vi "BusB Decoded Data Updated.vi"(8 "error in (no error)":errorcluster, 11 "BusB TypeDef":T1) -> (0 "error out":errorcluster)   [LabVIEW 2016, in "Impedance Data Acquisition and Decoding.lvlib"]
doc: "_____\nCreated using Delacor QMH Event Scripter 5.0.0.112."
uses:
  Impedance Data Acquisition and Decoding.lvlib
  BusB Typedef.ctl
  BusB Decoded Data Updated Argument--cluster.ctl
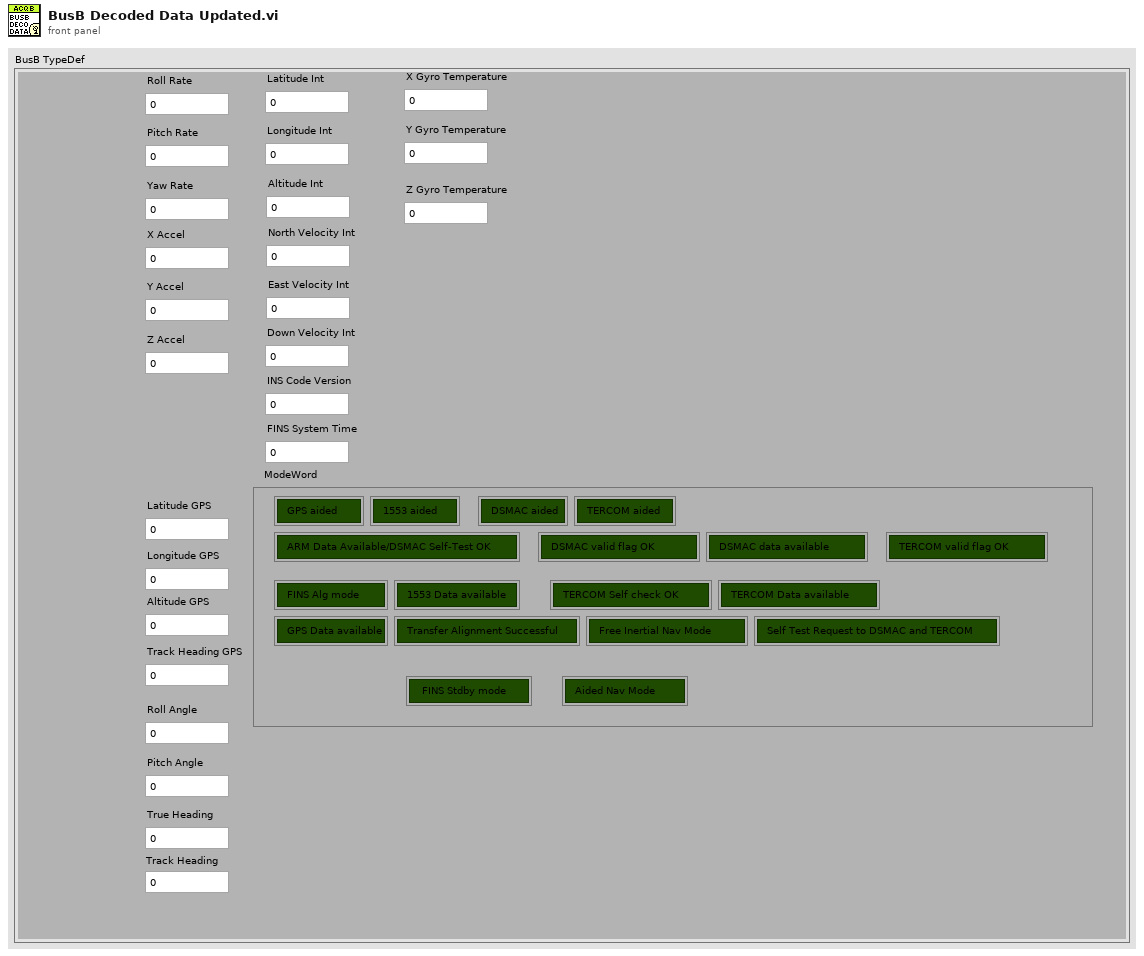
[diagram p1: front panel]
types:
  T1 = typedef "Impedance Data Acquisition and Decoding.lvlib/BusB Typedef.ctl" = cluster{"Pitch Rate":dbl, "Roll Rate":dbl, "Roll Angle":dbl, "Yaw Rate":dbl, "True Heading":dbl, "Pitch Angle":dbl, "Y Accel":dbl, "X Accel":dbl, "Z Accel":dbl, "X Gyro Temperature":dbl, "Longitude GPS":dbl, "Latitude GPS":dbl, "Altitude GPS":dbl, "Track Heading GPS":dbl, "Longitude Int":dbl, "Latitude Int":dbl, "Altitude Int":dbl, "FINS System Time":dbl, "East Velocity Int":dbl, "North Velocity Int":dbl, "INS Code Version":dbl, "ModeWord":cluster{"FINS Alg mode":bool, "GPS Data available":bool, "1553 Data available":bool, "Transfer Alignment Successful":bool, "TERCOM Self check OK":bool, "Free Inertial Nav Mode":bool, "TERCOM Data available":bool, "Self Test Request to DSMAC and TERCOM":bool, "ARM Data Available/DSMAC Self-Test OK":bool, "DSMAC valid flag OK":bool, "DSMAC data available":bool, "TERCOM valid flag OK":bool, "GPS aided":bool, "1553 aided":bool, "DSMAC aided":bool, "TERCOM aided":bool, "Aided Nav Mode":bool, " FINS Stdby mode":bool}, "Down Velocity Int":dbl, "Track Heading":dbl, "Y Gyro Temperature":dbl, "Z Gyro Temperature":dbl}
  T2 = typedef "Impedance Data Acquisition and Decoding.lvlib/BusB Decoded Data Updated Argument--cluster.ctl" = cluster{"BusB Decoded Data":T1}
  T3 = typedef "Impedance Data Acquisition and Decoding.lvlib/Broadcast Events--cluster.ctl" = cluster{"Module Did Init":refnum<user-event>, "Status Updated":refnum<user-event>, "Error Reported":refnum<user-event>, "Module Did Stop":refnum<user-event>, "Update Module Execution Status":refnum<user-event>, "Acquisition Stopped":refnum<user-event>, "BusB Raw Data":refnum<user-event>, "BusB Decoded Data Updated":refnum<user-event>, "Acquisition Started":refnum<user-event>, "Read Timeout Error Generation":refnum<user-event>}
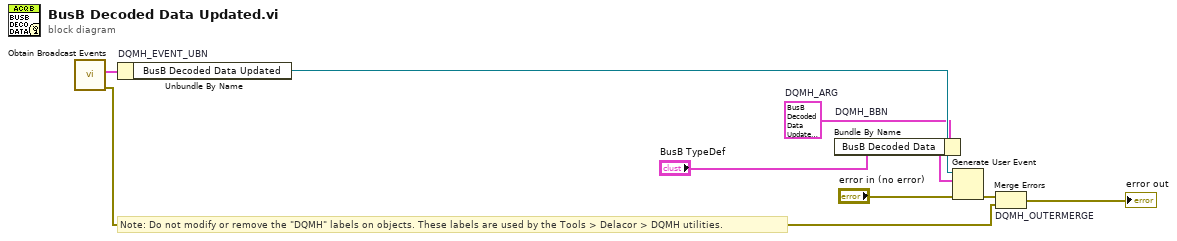
[diagram p0: block diagram]
diagram:
  w4 = T2 {"BusB Decoded Data"={"Pitch Rate"=0.0, "Roll Rate"=0.0, "Roll Angle"=0.0, "Yaw Rate"=0.0, "True Heading"=0.0, "Pitch Angle"=0.0, "Y Accel"=0.0, "X Accel"=0.0, "Z Accel"=0.0, "X Gyro Temperature"=0.0, "Longitude GPS"=0.0, "Latitude GPS"=0.0, "Altitude GPS"=0.0, "Track Heading GPS"=0.0, "Longitude Int"=0.0, "Latitude Int"=0.0, "Altitude Int"=0.0, "FINS System Time"=0.0, "East Velocity Int"=0.0, "North Velocity Int"=0.0, "INS Code Version"=0.0, "ModeWord"={"FINS Alg mode"=FALSE, "GPS Data available"=FALSE, "1553 Data available"=FALSE, "Transfer Alignment Successful"=FALSE, "TERCOM Self check OK"=FALSE, "Free Inertial Nav Mode"=FALSE, "TERCOM Data available"=FALSE, "Self Test Request to DSMAC and TERCOM"=FALSE, "ARM Data Available/DSMAC Self-Test OK"=FALSE, "DSMAC valid flag OK"=FALSE, "DSMAC data available"=FALSE, "TERCOM valid flag OK"=FALSE, "GPS aided"=FALSE, "1553 aided"=FALSE, "DSMAC aided"=FALSE, "TERCOM aided"=FALSE, "Aided Nav Mode"=FALSE, " FINS Stdby mode"=FALSE}, "Down Velocity Int"=0.0, "Track Heading"=0.0, "Y Gyro Temperature"=0.0, "Z Gyro Temperature"=0.0}}  # DQMH_ARG
  # "Note: Do not modify or remove the \"DQMH\" labels on objects. These labels are used by the Tools > Delacor > DQMH utilities."
  n1 = call "Obtain Broadcast Events.vi"() -> ("error out"=w3:errorcluster, "FINS3-E BusB Data Acquisition and Decoding Broadcast Events"=w2:T3)  [unwired: 10 in]
  n2 = Unbundle By Name "DQMH_EVENT_UBN"(w2) -> ("BusB Decoded Data Updated"=w6:refnum<user-event>)
  n3 = Bundle By Name "DQMH_BBN"(cluster=w4, "BusB Decoded Data"="BusB TypeDef") -> (w7:T2)
  n4 = Generate User Event(user event=w6, event data cluster=w7, error in="error in (no error)") -> (error out=w5:errorcluster)  [unwired: 1 in, 1 out]
  n5 = Merge Errors "DQMH_OUTERMERGE"(w5, w3) -> (→"error out":errorcluster)
